vi "StringTag.write_lua.vi"(5 "LuaVIEW reference":T1) -> (15 "error out":errorcluster)   [LabVIEW 2012]
doc: "Write a string with the given value and an optional timestamp to a string tag. Note that there are no restrictions on the content so that it can be used to store arbitrary data. The only limitation is that the string should fit comfortably in memory since the most recently written strings are buffered in-memory for each tag.\n\nBeware that this function is likely to cause immediate disk access: the strings are stored in a separate file per tag which will be appended to when the string being written does not equal either a recently written string that is still buffered in memory, an empty string, or the special string \"UNDEFINED\". The frequency with which novel strings can be written to multiple string tags will therefore be limited by the seek period of the head of the harddisk on which the logging database is stored.\n\nTo apply the timestamp and later be able to retrieve the string, a point with the specified or current time is logged with a value equal to the byte offset in the strings file at which the string was stored. These points are subject to buffering, aggregation, and flushing in the very same manner as points of numerical tags. The \"UNDEFINED\" string is specified via the special NaN point value and serves the same purpose as NaN values of numerical tags.\n\nTimestamps of subsequently written strings may not decrease. When no timestamp is specified, the time in seconds since the LabVIEW epoch (1-Jan-1904) as obtained via the \"Library Time.vi\" is used. This VI exists to allow custom time sources. Its default implementation simply calls \"Get Date/Time In Seconds\" LabVIEW node, which in turn obtains its time from the system clock. Beware that the system clock has a platform dependent resolution and will drift unless corrected for, e.g. using the ntp protocol.\nParameters:\nobj:strtag\nstr:value, string value to write.\n[num:time], optional timestamp, when omitted the current time is used.\nErrors:\nDead or invalid tag object.\nData logger not initialized."
uses:
  luaview/typedefs/t_LuaVIEW Reference.ctl
  luaview/subvis/private/LuaVIEW Pull (object).vi
  luaview/subvis/private/LuaVIEW Pull (string).vi
  luaview/subvis/private/LuaVIEW Pull (number).vi
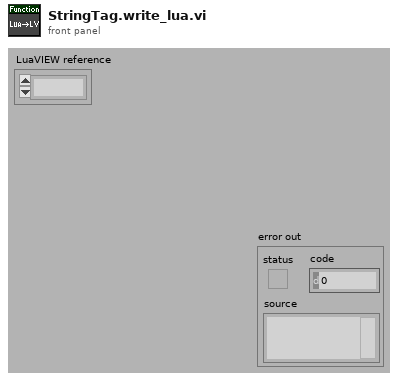
[diagram p1: front panel]
types:
  T1 = typedef "t_LuaVIEW Reference.ctl" = refnum<k1>
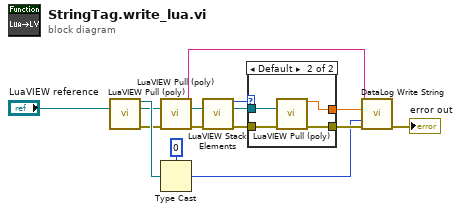
[diagram p0: block diagram]
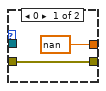
[diagram p2: hidden frame]
diagram:
  n1 = call-poly "LuaVIEW Pull (poly).vi"("LuaVIEW reference in"="LuaVIEW reference") -> ("object refnum"=w15:refnum<vi>, "LuaVIEW reference out"=w12:T1, "error out"=w13:errorcluster)  [unwired: 11 in, 1 out]
  n2 = call-poly "LuaVIEW Pull (poly).vi"("LuaVIEW reference in"=w12, "error in (no error)"=w13) -> ("string"=w1:string, "LuaVIEW reference out"=w9:T1, "error out"=w10:errorcluster)  [unwired: 11 in]
  n3 = Type Cast(type=0 ("read index in"), x=w15) -> (*(type *) &x=w4:i32)
  n4 = call "LuaVIEW Stack Elements.vi"("LuaVIEW reference in"=w9, "error in (no error)"=w10) -> ("elements"=w8:i32, "LuaVIEW reference out"=w7:T1, "error out"=w6:errorcluster)  [unwired: 11 in]
  n5 = case shown="Default" w8 {
    tunnel: [w17 w21] -> w5
    tunnel: [nan ("number") w20] -> w2
    tunnel: w7 -> [_ w19]
    tunnel: w6 -> [w17 w18]
    frame 0 {
    }
    frame Default {
      n6 = call-poly "LuaVIEW Pull (poly).vi"("LuaVIEW reference in"=w19, "error in (no error)"=w18) -> ("number"=w20:dbl, "error out"=w21:errorcluster)  [unwired: 11 in, 1 out]
    }
  }
  n7 = call "DataLog Write String.vi"("string"=w1, "time (current)"=w2, "tag index in (use tag)"=w4, "error in (no error)"=w5) -> ("error out"=→"error out":errorcluster)  [unwired: 10 in, 1 out]
